vi "Example.vi"() -> ()   [LabVIEW 2023]
panel:
  in  "Stop Streaming":bool
  out "Vedeo":T1(plugin-control)
  out "Stop Capture Success":bool
  out "Start Capture Success":bool
  out "Close_Completed":bool
  out "Signal Status":T2
  out "Open_Device_Completed":bool
  out "Initialize Success":bool
  in  "error in":errorcluster
  out "error out":errorcluster
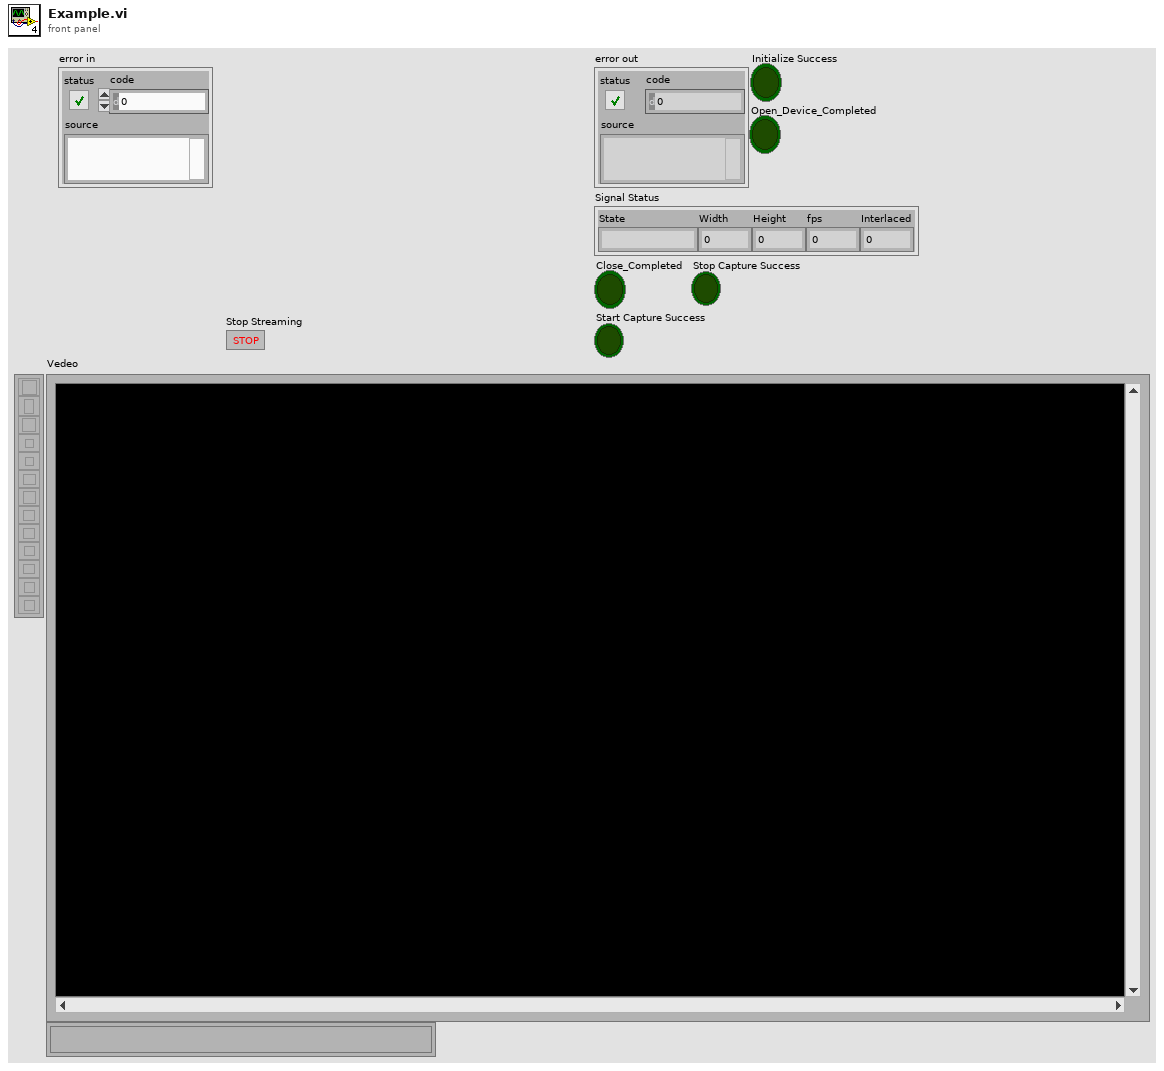
[diagram p1: front panel]
types:
  T1 = typedef "IMAQ Image.ctl" = refnum<image>
  T2 = cluster{"State":string, "Width":i32, "Height":i32, "fps":i32, "Interlaced":i32}
  T3 = typedef "Image Type" = u32
  T4 = cluster{"Width":i32, "Height":i32, "Channel":i32}
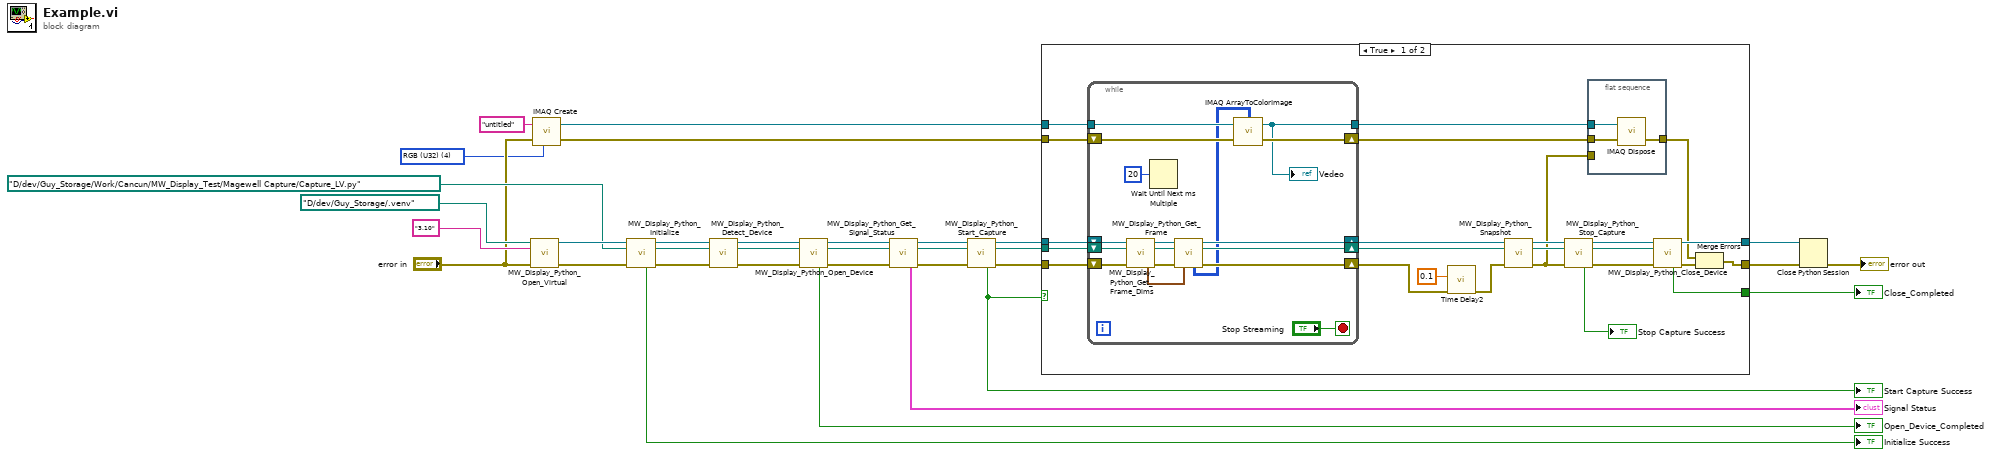
[diagram p0: block diagram]
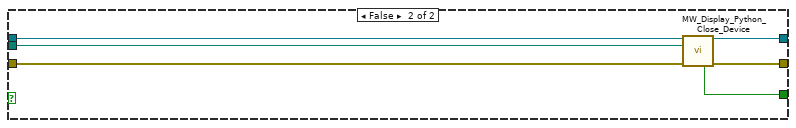
[diagram p2: hidden frame]
diagram:
  w4 = T3 4 items=["Grayscale (U8)", "Grayscale (I16)", "Grayscale (SGL)", "Complex (CSG)", "RGB (U32)", "HSL (U32)", "RGB (U64)", "Grayscale (U16)"] ("Image Type")
  n1 = call "MW_Display_Python_Open_Virtual.vi"("Env path"=path "D:/dev/Guy_Storage/.venv", "Python version"="3.10", "error in"="error in") -> ("session out"=w32:refnum<k35>, "error out"=w33:errorcluster)  [unwired: 11 in]
  n2 = call "IMAQ Create"("Image Name"="untitled", "Image Type"=w4, "error in (no error)"="error in") -> ("New Image"=w2:T1, "error out"=w3:errorcluster)  [unwired: 2 in]
  n3 = call "MW_Display_Python_Initialize.vi"("session in"=w32, "module path"=path "D:/dev/Guy_Storage/Work/Cancun/MW_Display_Test/Magewell Capture/Capture_LV.py", "error in"=w33) -> ("session out"=w25:refnum<k35>, "module path out"=w24:path, "Initialize Success"=→"Initialize Success":bool, "error out"=w26:errorcluster)  [unwired: 9 in]
  n4 = call "MW_Display_Python_Detect_Device.vi"("session in"=w25, "module path"=w24, "error in"=w26) -> ("session out"=w22:refnum<k35>, "module path out"=w21:path, "error out"=w23:errorcluster)  [unwired: 8 in, 2 out]
  n5 = call "MW_Display_Python_Open_Device.vi"("session in"=w22, "module path"=w21, "error in"=w23) -> ("session out"=w18:refnum<k35>, "module path out"=w17:path, "Open_Device_Completed"=→"Open_Device_Completed":bool, "error out"=w19:errorcluster)  [unwired: 9 in]
  n6 = call "MW_Display_Python_Get_Signal_Status.vi"("session in"=w18, "module path"=w17, "error in"=w19) -> ("session out"=w14:refnum<k35>, "module path out"=w13:path, "Signal Status"=→"Signal Status":T2, "error out"=w15:errorcluster)  [unwired: 9 in]
  n7 = call "MW_Display_Python_Start_Capture.vi"("session in"=w14, "module path"=w13, "error in"=w15) -> ("session out"=w11:refnum<k35>, "module path out"=w10:path, "Start Capture Success"=w6:bool, "error out"=w12:errorcluster)  [unwired: 9 in]
  "Start Capture Success" <- w6
  n8 = case shown="True" w6 {
    tunnel: w12 -> [w54 w83]
    tunnel: w11 -> [w53 w82]
    tunnel: w10 -> [w52 w81]
    tunnel: [w57 w80] -> w9
    tunnel: [w36 w79] -> w8
    tunnel: [w55 w78] -> w7
    tunnel: w3 -> [w40 _]
    tunnel: w2 -> [w39 _]
    frame True {
      n9 = while {
        shift-right: [w71] -> w43
        shift-left: w54 -> [w77]
        shift-right: [w70] -> w42
        shift-left: w53 -> [w76]
        shift-right: [w69] -> w41
        shift-left: w52 -> [w75]
        tunnel: w39 -> [w66]
        shift-right: [w65] -> w38
        shift-left: w40 -> [w67]
        tunnel: [w63] -> w37
        stop <- "Stop Streaming" stop-if-true
        n10 = call "MW_Display_Python_Get_Frame_Dims.vi"("session in"=w76, "module path"=w75, "error in"=w77) -> ("session out"=w73:refnum<k35>, "module path out"=w72:path, "Frame Dims"=w68:T4, "error out"=w74:errorcluster)  [unwired: 9 in]
        n11 = Wait Until Next ms Multiple(millisecond multiple=u32 20) -> ()  [unwired: 1 out]
        n12 = call "MW_Display_Python_Get_Frame.vi"("session in"=w73, "module path"=w72, "error in"=w74, "Frame Dims"=w68) -> ("session out"=w70:refnum<k35>, "module path out"=w69:path, "RGB Pixels"=w64:u32[][], "error out"=w71:errorcluster)  [unwired: 8 in]
        n13 = call "IMAQ ArrayToColorImage"("Image Pixels (U32)"=w64, "Image"=w66, "error in (no error)"=w67) -> ("Image Out"=w63:T1, "error out"=w65:errorcluster)  [unwired: 2 in]
        "Vedeo" <- w63
      }
      n14 = call "Time Delay2"("error in (no error)"=w43, "Delay Time (s)"=0.1) -> ("error out"=w45:errorcluster)  [unwired: 9 in]
      n15 = call "MW_Display_Python_Snapshot.vi"("session in"=w42, "module path"=w41, "error in"=w45) -> ("session out"=w46:refnum<k35>, "module path out"=w47:path, "error out"=w34:errorcluster)  [unwired: 10 in]
      n16 = call "MW_Display_Python_Stop_Capture.vi"("session in"=w46, "module path"=w47, "error in"=w34) -> ("session out"=w50:refnum<k35>, "module path out"=w49:path, "Stop Capture Success"=→"Stop Capture Success":bool, "error out"=w51:errorcluster)  [unwired: 9 in]
      n17 = flat-sequence {
        tunnel: w38 -> [w60]
        tunnel: w37 -> [w59]
        tunnel: [w58] -> w35
        tunnel: w34 -> [_]
        frame #0 {
          n18 = call "IMAQ Dispose"("Image"=w59, "error in (no error)"=w60) -> ("error out"=w58:errorcluster)  [unwired: 4 in]
        }
      }
      n19 = call "MW_Display_Python_Close_Device.vi"("session in"=w50, "module path"=w49, "error in"=w51) -> ("session out"=w57:refnum<k35>, "Close_Completed"=w55:bool, "error out"=w56:errorcluster)  [unwired: 9 in, 1 out]
      n20 = Merge Errors(w35, w56) -> (w36:errorcluster)
    }
    frame False {
      n21 = call "MW_Display_Python_Close_Device.vi"("session in"=w82, "module path"=w81, "error in"=w83) -> ("session out"=w80:refnum<k35>, "Close_Completed"=w78:bool, "error out"=w79:errorcluster)  [unwired: 9 in, 1 out]
    }
  }
  "Close_Completed" <- w7
  n22 = Close Python Session(session in=w9, error in=w8) -> (11:→"error out":errorcluster)
